vi "Sample Data Demo v1.vi"() -> ()   [LabVIEW 2020]
doc: "Sample data demonstration, also allows to test saving functinoality without having to be conected to the machine."
panel:
  out "output cluster 3":cluster{dbl[], dbl[]}
  out "output cluster":cluster{dbl[], dbl[]}
  in  "Tab Control":enum32{"A-Scan", "B-Scan", "C-Scan"}(tab)
  out "A-Scan":cluster{dbl[], dbl[]}(graph)
  in  "Folder to Save Data":path
  in  "File Name":string
  in  "Confirm Saving Options":bool
  in  "A Scan Scan":bool
  in  "Desired 'Y' Position":dbl
  in  "Desired 'X' Position":dbl
  in  "File Format":T1(radio)
  in  "B-Scan File Name":string
  in  "Folder to Save B-Scan Data":path
  out "B-Scan":dbl[][](graph)
  in  "Depth Along Axis":dbl
  in  "Position of Selected Axis":dbl
  in  "B Scan Scan":bool
  in  "Confirm Saving Options 2":bool
  in  "File Format":T1(radio)
  in  "Folder To Save A-Scan Data":path
  in  "A-Scan File Name":string
  in  "B-Scan Build Up Quality":T2(radio)
  in  "C-Scan Build Up Quantity":T2(radio)
  in  "Total 'Y' Distance to Cover":dbl
  in  "Total 'X' Distance to Cover":dbl
  in  "C Scan Scan":bool
  out "C-Scan":dbl[][](graph)
  in  "File Format":T1(radio)=enum."Do Not Save"
  in  "Confirm Saving Options":bool
  in  "A-Scan File Name":string
  in  "Folder to Save A-Scan Data":path
  in  "Folder to Save C-Scan Data":path
  in  "C-Scan File Name":string
  # "Scan Parameters"
  # "Saving Options"
  # "Scan Parameters"
  # "Saving Options"
  # "Scan Parameters"
  # "Saving Options"
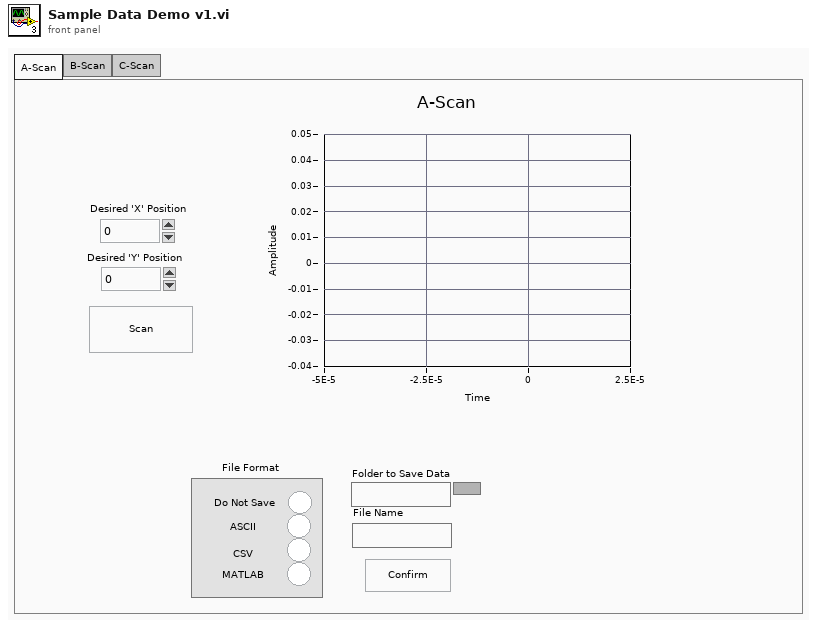
[diagram p1: front panel]
types:
  T1 = enum32{"No Selection", "Do Not Save", "ASCII", "CSV", "MATLAB"}
  T2 = enum32{"No Selection", "Peak Positive", "Peak Negative", "Peak Magnitude", "Energy"}
  T3 = enum16{"open", "replace", "create", "open or create", "replace or create", "replace or create with confirmation"}
  T4 = enum8{"Enabled", "Disabled", "Disabled and Grayed Out"}
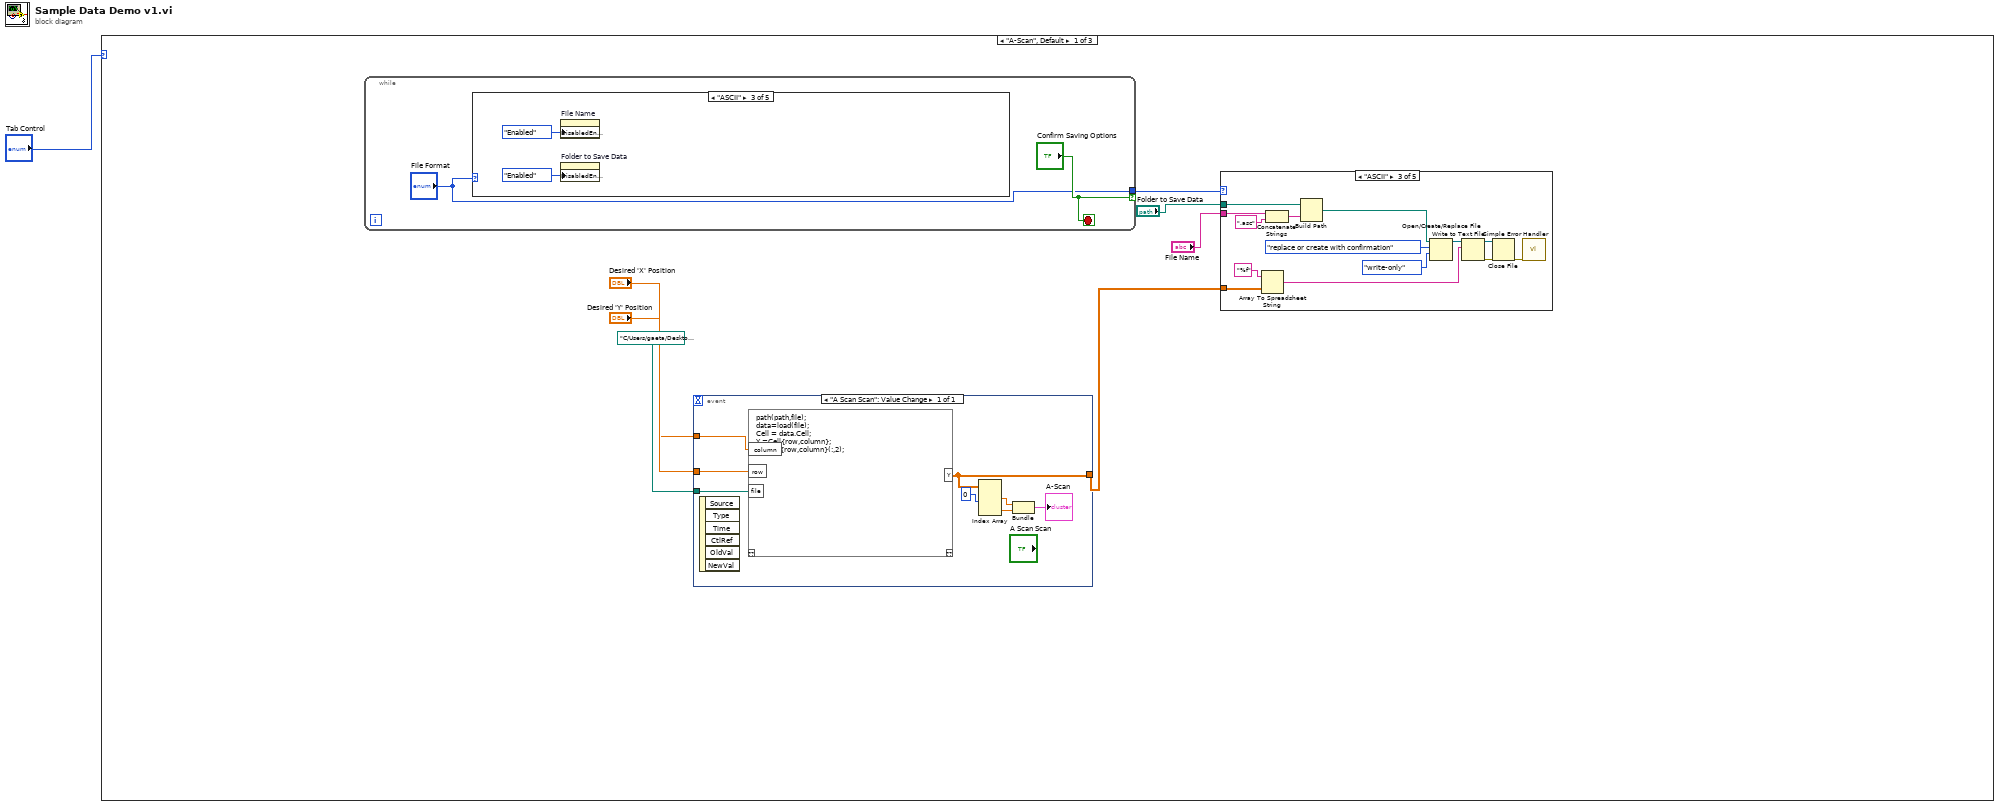
[diagram p0: block diagram]
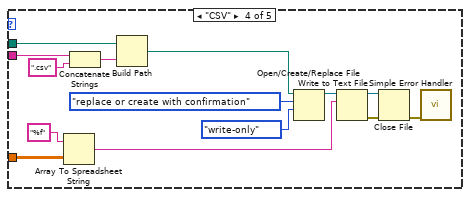
[diagram p4: hidden frame]
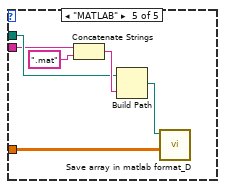
[diagram p5: hidden frame]
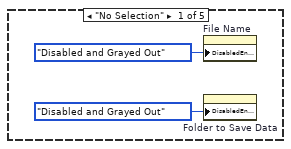
[diagram p6: hidden frame]
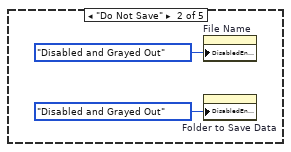
[diagram p7: hidden frame]
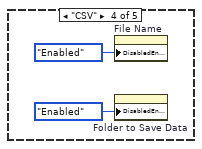
[diagram p8: hidden frame]
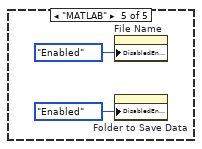
[diagram p9: hidden frame]
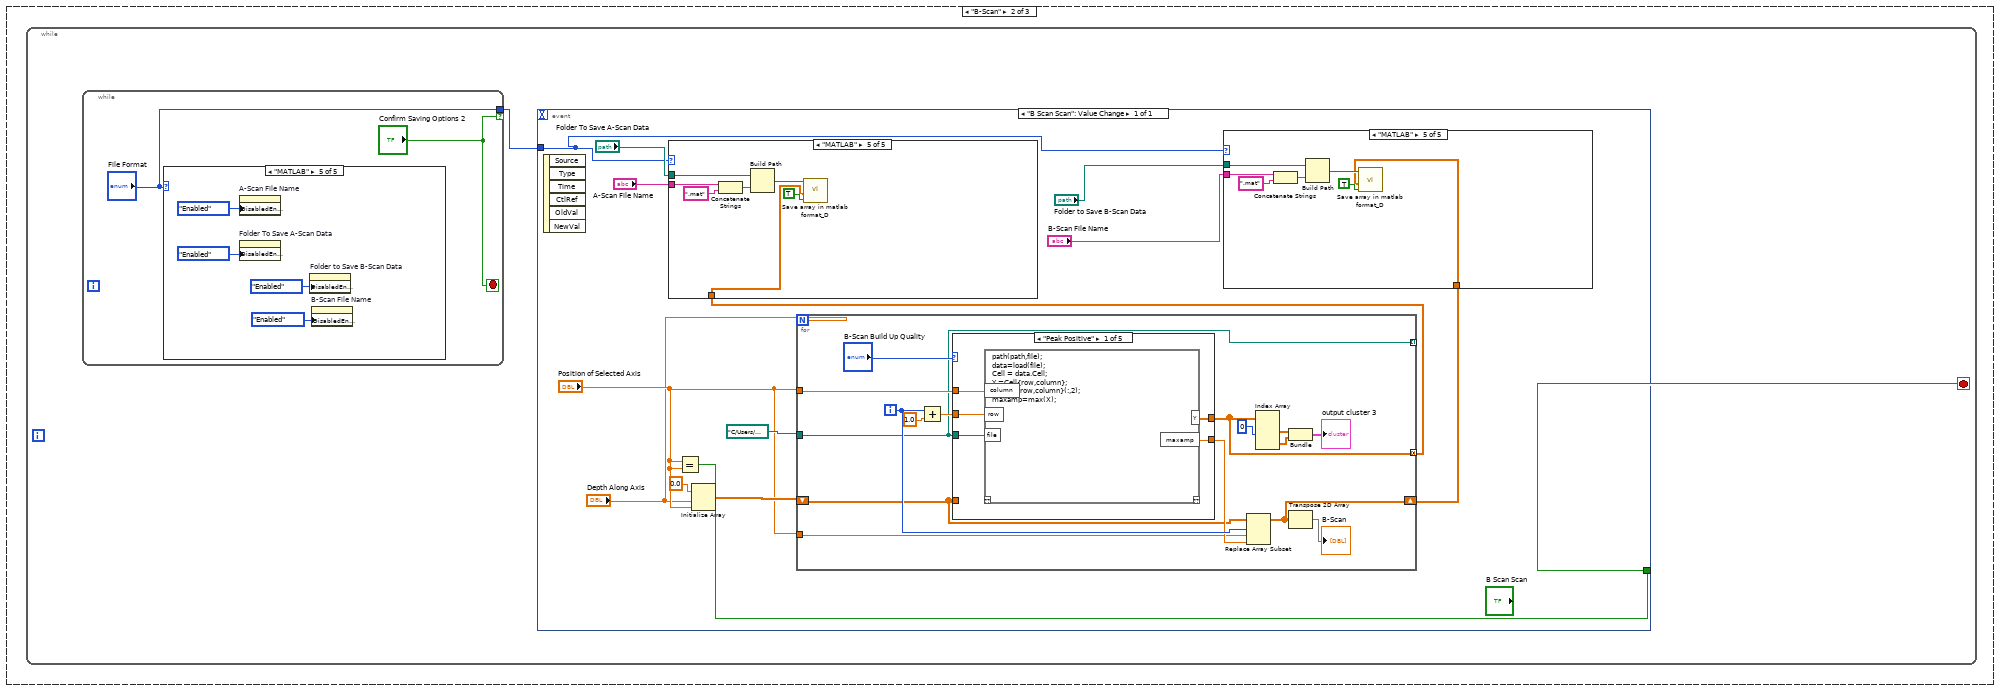
[diagram p10: hidden frame]
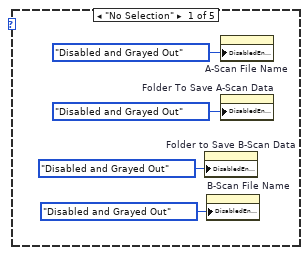
[diagram p11: hidden frame]
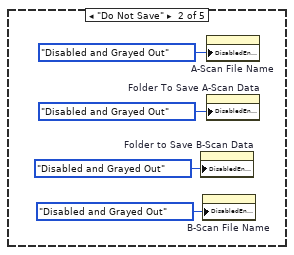
[diagram p12: hidden frame]
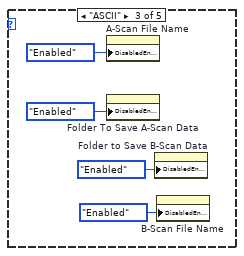
[diagram p13: hidden frame]
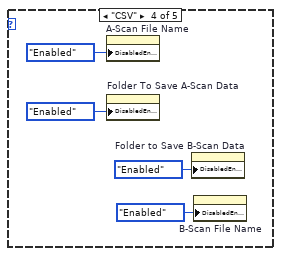
[diagram p14: hidden frame]
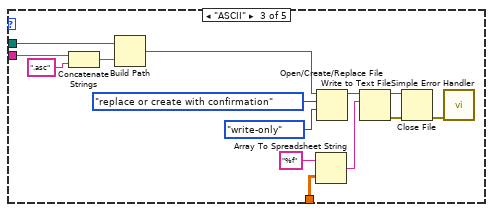
[diagram p17: hidden frame]
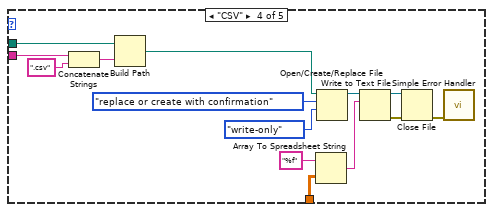
[diagram p18: hidden frame]
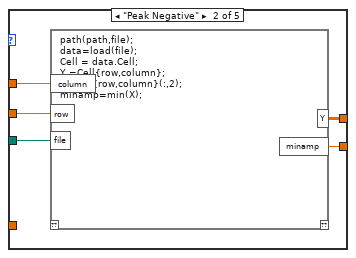
[diagram p19: hidden frame]
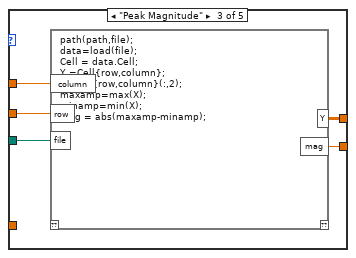
[diagram p20: hidden frame]
diagram:
  n1 = case shown="\"A-Scan\", Default" "Tab Control" {
    frame "A-Scan", Default {
      n2 = while {
        tunnel: ["File Format"] -> w2 if="Confirm Saving Options"
        stop <- "Confirm Saving Options" stop-if-true
        n3 = case shown="\"ASCII\"" "File Format" {
          frame "No Selection" {
            n4 = property on="File Name" class="Str"("DisabledEnum"=T4."Disabled and Grayed Out" ("Disabled")) -> ()  [unwired: 2 in, 2 out]
            n5 = property on="Folder to Save Data" class="Path"("DisabledEnum"=T4."Disabled and Grayed Out" ("Disabled")) -> ()  [unwired: 2 in, 2 out]
          }
          frame "Do Not Save" {
            n6 = property on="File Name" class="Str"("DisabledEnum"=T4."Disabled and Grayed Out" ("Disabled")) -> ()  [unwired: 2 in, 2 out]
            n7 = property on="Folder to Save Data" class="Path"("DisabledEnum"=T4."Disabled and Grayed Out" ("Disabled")) -> ()  [unwired: 2 in, 2 out]
          }
          frame "ASCII" {
            n8 = property on="File Name" class="Str"("DisabledEnum"=T4."Enabled" ("Disabled")) -> ()  [unwired: 2 in, 2 out]
            n9 = property on="Folder to Save Data" class="Path"("DisabledEnum"=T4."Enabled" ("Disabled")) -> ()  [unwired: 2 in, 2 out]
          }
          frame "CSV" {
            n10 = property on="File Name" class="Str"("DisabledEnum"=T4."Enabled" ("Disabled")) -> ()  [unwired: 2 in, 2 out]
            n11 = property on="Folder to Save Data" class="Path"("DisabledEnum"=T4."Enabled" ("Disabled")) -> ()  [unwired: 2 in, 2 out]
          }
          frame "MATLAB" {
            n12 = property on="File Name" class="Str"("DisabledEnum"=T4."Enabled" ("Disabled")) -> ()  [unwired: 2 in, 2 out]
            n13 = property on="Folder to Save Data" class="Path"("DisabledEnum"=T4."Enabled" ("Disabled")) -> ()  [unwired: 2 in, 2 out]
          }
        }
      }
      n14 = event shown="[0] \"A Scan Scan\": Value Change" {
        selector: _ -> [_]
        dyn-events: _ -> [_]
        timeout: _ -> [_]
        tunnel: "Desired 'X' Position" -> [w56]
        tunnel: "Desired 'Y' Position" -> [w58]
        tunnel: path "C:/Users/gaeta/Desktop/Unif Leerstof/Individual Project/Osc. Data/wetransfer-86c2d3/2DZXaxisscan 0.28MHz 30x30mm 20mvpp 1020L centre 390mm from td plane.mat" ("Input Data Path") -> [w57]
        tunnel: [w55] -> w5
        event "A Scan Scan": Value Change {
          n15 = event-data() -> ()  [unwired: 1 in, 6 out]
          n16 = script code="path(path,file);\ndata=load(file);\nCell = data.Cell;\nY =Cell{row,column};\nX=Cell{row,column}(:,2);"("row"=w58, "file"=w57, "column"=w56) -> ("Y"=w55:dbl[][])  [unwired: 1 in, 1 out]
          n17 = Index Array(array=w55, index (col) #1=0 ("disabled index (col)")) -> (element #1=w61:dbl[], element #2=w60:dbl[])  [unwired: 3 in]
          n18 = Bundle(w61, w60) -> (→"A-Scan":cluster{dbl[], dbl[]})  [unwired: 1 in]
        }
      }
      n19 = case shown="\"ASCII\"" w2 {
        tunnel: w5 -> [_ _ w9 w25 w37]
        tunnel: "Folder to Save Data" -> [_ _ w11 w24 w39]
        tunnel: "File Name" -> [_ _ w10 w23 w38]
        frame "No Selection" {
        }
        frame "Do Not Save" {
        }
        frame "ASCII" {
          n20 = Array To Spreadsheet String(array=w9, 3:"%f" ("format string")) -> (spreadsheet string=w21:string)  [unwired: 1 in]
          n21 = Concatenate Strings(w10, ".asc" ("string")) -> (w16:string)
          n22 = Build Path(base path=w11, name or relative path=w16) -> (appended path=w17:path)
          n23 = Open/Create/Replace File(file path (use dialog)=w17, operation (0:open)=T3."replace or create with confirmation", access (0:read/write)=enum16{"read/write", "read-only", "write-only"}."write-only") -> (refnum out=w22:refnum<file>)  [unwired: 1 in, 4 out]
          n24 = Write to Text File(file (use dialog)=w22, text=w21) -> (refnum out=w20:refnum<file>, error out=w19:errorcluster)  [unwired: 2 in, 1 out]
          n25 = Close File(refnum=w20, error in=w19) -> (error out=w18:errorcluster)  [unwired: 1 out]
          n26 = call <vilib>:"Simple Error Handler.vi"("error in (no error)"=w18) -> ()  [unwired: 1 in, 8 out]
        }
        frame "CSV" {
          n27 = Array To Spreadsheet String(array=w25, 3:"%f" ("format string")) -> (spreadsheet string=w32:string)  [unwired: 1 in]
          n28 = Concatenate Strings(w23, ".csv" ("string")) -> (w31:string)
          n29 = Build Path(base path=w24, name or relative path=w31) -> (appended path=w30:path)
          n30 = Open/Create/Replace File(file path (use dialog)=w30, operation (0:open)=T3."replace or create with confirmation", access (0:read/write)=enum16{"read/write", "read-only", "write-only"}."write-only") -> (refnum out=w36:refnum<file>)  [unwired: 1 in, 4 out]
          n31 = Write to Text File(file (use dialog)=w36, text=w32) -> (refnum out=w33:refnum<file>, error out=w34:errorcluster)  [unwired: 2 in, 1 out]
          n32 = Close File(refnum=w33, error in=w34) -> (error out=w35:errorcluster)  [unwired: 1 out]
          n33 = call <vilib>:"Simple Error Handler.vi"("error in (no error)"=w35) -> ()  [unwired: 1 in, 8 out]
        }
        frame "MATLAB" {
          n34 = Concatenate Strings(w38, ".mat" ("string")) -> (w41:string)
          n35 = Build Path(base path=w39, name or relative path=w41) -> (appended path=w42:path)
          n36 = call "Save array in matlab format_D"("2D array"=w37, "file path (dialog if empty)"=w42) -> ()  [unwired: 5 in, 1 out]
        }
      }
    }
    frame "B-Scan" {
      n37 = while {
        stop <- w64 stop-if-true
        n38 = while {
          tunnel: ["File Format"] -> w63 if="Confirm Saving Options 2"
          stop <- "Confirm Saving Options 2" stop-if-true
          n39 = case shown="\"MATLAB\"" "File Format" {
            frame "No Selection" {
              n40 = property on="Folder to Save B-Scan Data" class="Path"("DisabledEnum"=T4."Disabled and Grayed Out" ("Disabled")) -> ()  [unwired: 2 in, 2 out]
              n41 = property on="B-Scan File Name" class="Str"("DisabledEnum"=T4."Disabled and Grayed Out" ("Disabled")) -> ()  [unwired: 2 in, 2 out]
              n42 = property on="A-Scan File Name" class="Str"("DisabledEnum"=T4."Disabled and Grayed Out" ("Disabled")) -> ()  [unwired: 2 in, 2 out]
              n43 = property on="Folder To Save A-Scan Data" class="Path"("DisabledEnum"=T4."Disabled and Grayed Out" ("Disabled")) -> ()  [unwired: 2 in, 2 out]
            }
            frame "Do Not Save" {
              n44 = property on="Folder to Save B-Scan Data" class="Path"("DisabledEnum"=T4."Disabled and Grayed Out" ("Disabled")) -> ()  [unwired: 2 in, 2 out]
              n45 = property on="B-Scan File Name" class="Str"("DisabledEnum"=T4."Disabled and Grayed Out" ("Disabled")) -> ()  [unwired: 2 in, 2 out]
              n46 = property on="A-Scan File Name" class="Str"("DisabledEnum"=T4."Disabled and Grayed Out" ("Disabled")) -> ()  [unwired: 2 in, 2 out]
              n47 = property on="Folder To Save A-Scan Data" class="Path"("DisabledEnum"=T4."Disabled and Grayed Out" ("Disabled")) -> ()  [unwired: 2 in, 2 out]
            }
            frame "ASCII" {
              n48 = property on="A-Scan File Name" class="Str"("DisabledEnum"=T4."Enabled" ("Disabled")) -> ()  [unwired: 2 in, 2 out]
              n49 = property on="Folder To Save A-Scan Data" class="Path"("DisabledEnum"=T4."Enabled" ("Disabled")) -> ()  [unwired: 2 in, 2 out]
              n50 = property on="Folder to Save B-Scan Data" class="Path"("DisabledEnum"=T4."Enabled" ("Disabled")) -> ()  [unwired: 2 in, 2 out]
              n51 = property on="B-Scan File Name" class="Str"("DisabledEnum"=T4."Enabled" ("Disabled")) -> ()  [unwired: 2 in, 2 out]
            }
            frame "CSV" {
              n52 = property on="A-Scan File Name" class="Str"("DisabledEnum"=T4."Enabled" ("Disabled")) -> ()  [unwired: 2 in, 2 out]
              n53 = property on="Folder To Save A-Scan Data" class="Path"("DisabledEnum"=T4."Enabled" ("Disabled")) -> ()  [unwired: 2 in, 2 out]
              n54 = property on="Folder to Save B-Scan Data" class="Path"("DisabledEnum"=T4."Enabled" ("Disabled")) -> ()  [unwired: 2 in, 2 out]
              n55 = property on="B-Scan File Name" class="Str"("DisabledEnum"=T4."Enabled" ("Disabled")) -> ()  [unwired: 2 in, 2 out]
            }
            frame "MATLAB" {
              n56 = property on="A-Scan File Name" class="Str"("DisabledEnum"=T4."Enabled" ("Disabled")) -> ()  [unwired: 2 in, 2 out]
              n57 = property on="Folder To Save A-Scan Data" class="Path"("DisabledEnum"=T4."Enabled" ("Disabled")) -> ()  [unwired: 2 in, 2 out]
              n58 = property on="Folder to Save B-Scan Data" class="Path"("DisabledEnum"=T4."Enabled" ("Disabled")) -> ()  [unwired: 2 in, 2 out]
              n59 = property on="B-Scan File Name" class="Str"("DisabledEnum"=T4."Enabled" ("Disabled")) -> ()  [unwired: 2 in, 2 out]
            }
          }
        }
        n60 = event shown="[0] \"B Scan Scan\": Value Change" {
          selector: _ -> [_]
          dyn-events: _ -> [_]
          timeout: _ -> [_]
          tunnel: [w92] -> w64
          tunnel: w63 -> [w87]
          event "B Scan Scan": Value Change {
            n61 = event-data() -> ()  [unwired: 1 in, 6 out]
            n62 = Equal?(x="Position of Selected Axis", y="Position of Selected Axis") -> (x = y?=w92:bool)
            n63 = Initialize Array(0.0 ("element"), "Depth Along Axis", "Position of Selected Axis") -> (w95:dbl[][])
            n64 = for {
              N: "Depth Along Axis" -> [_]
              tunnel: [w136] -> _ mode=indexing
              tunnel: "Position of Selected Axis" -> [w144]
              shift-right: [w145] -> w88
              shift-left: w95 -> [w141]
              tunnel: [w137] -> w93 mode=concatenating
              tunnel: path "C:/Users/gaeta/Desktop/Unif Leerstof/Individual Project/Osc. Data/wetransfer-86c2d3/2DZXaxisscan 0.28MHz 30x30mm 20mvpp 1020L centre 390mm from td plane.mat" ("Input Data Path") -> [w136]
              tunnel: "Position of Selected Axis" -> [w135]
              i -> [w146]
              n65 = Add(x=w146, y=1.0) -> (x+y=w143:dbl)
              n66 = case shown="\"Peak Positive\"" "B-Scan Build Up Quality" {
                tunnel: w144 -> [w151 w156 w161 w166 _]
                tunnel: w143 -> [w155 w160 w163 w168 _]
                tunnel: w136 -> [w154 w159 w162 w167 _]
                tunnel: [w152 w158 w164 w169 _] -> w142
                tunnel: [w153 w157 w165 w170 _] -> w137
                tunnel: w141 -> [_ _ _ _ _]
                frame "Peak Positive" {
                  n67 = script code="path(path,file);\ndata=load(file);\nCell = data.Cell;\nY =Cell{row,column};\nX=Cell{row,column}(:,2);\nmaxamp=max(X);"("row"=w155, "file"=w154, "column"=w151) -> ("Y"=w153:dbl[][], "maxamp"=w152:dbl)  [unwired: 1 in, 1 out]
                }
                frame "Peak Negative" {
                  n68 = script code="path(path,file);\ndata=load(file);\nCell = data.Cell;\nY =Cell{row,column};\nX=Cell{row,column}(:,2);\nminamp=min(X);"("row"=w160, "file"=w159, "column"=w156) -> ("Y"=w157:dbl[][], "minamp"=w158:dbl)  [unwired: 1 in, 1 out]
                }
                frame "Peak Magnitude" {
                  n69 = script code="path(path,file);\ndata=load(file);\nCell = data.Cell;\nY =Cell{row,column};\nX=Cell{row,column}(:,2);\nmaxamp=max(X);\nminamp=min(X);\nmag = abs(maxamp-minamp);"("row"=w163, "file"=w162, "column"=w161) -> ("Y"=w165:dbl[][], "mag"=w164:dbl)  [unwired: 1 in, 1 out]
                }
                frame "Energy" {
                  n70 = script code="path(path,file);\ndata=load(file);\nCell = data.Cell;\nY =Cell{row,column};\nX=Cell{row,column}(:,2);\narea=trapz(X);"("row"=w168, "file"=w167, "column"=w166) -> ("Y"=w170:dbl[][], "area"=w169:dbl)  [unwired: 1 in, 1 out]
                }
                frame "No Selection" {
                }
              }
              n71 = Replace Array Subset(array=w141, new element=w142, index (row)=w146, index (col)=w135) -> (w145:dbl[][])
              n72 = Index Array(array=w137, index (col) #1=0 ("disabled index (col)")) -> (element #1=w148:dbl[], element #2=w149:dbl[])  [unwired: 3 in]
              n73 = Bundle(w148, w149) -> (→"output cluster 3":cluster{dbl[], dbl[]})  [unwired: 1 in]
              n74 = Transpose 2D Array(2D array=w145) -> (transposed array=→"B-Scan":dbl[][])
            }
            n75 = case shown="\"MATLAB\"" w87 {
              tunnel: "Folder To Save A-Scan Data" -> [_ _ w173 w187 w202]
              tunnel: "A-Scan File Name" -> [_ _ w172 w186 w201]
              tunnel: w93 -> [_ _ w171 w185 w199]
              frame "No Selection" {
              }
              frame "Do Not Save" {
              }
              frame "ASCII" {
                n76 = Concatenate Strings(w172, ".asc" ("string")) -> (w178:string)
                n77 = Build Path(base path=w173, name or relative path=w178) -> (appended path=w179:path)
                n78 = Array To Spreadsheet String(array=w171, 3:"%f" ("format string")) -> (spreadsheet string=w183:string)  [unwired: 1 in]
                n79 = Open/Create/Replace File(file path (use dialog)=w179, operation (0:open)=T3."replace or create with confirmation", access (0:read/write)=enum16{"read/write", "read-only", "write-only"}."write-only") -> (refnum out=w184:refnum<file>)  [unwired: 1 in, 4 out]
                n80 = Write to Text File(file (use dialog)=w184, text=w183) -> (refnum out=w182:refnum<file>, error out=w181:errorcluster)  [unwired: 2 in, 1 out]
                n81 = Close File(refnum=w182, error in=w181) -> (error out=w180:errorcluster)  [unwired: 1 out]
                n82 = call <vilib>:"Simple Error Handler.vi"("error in (no error)"=w180) -> ()  [unwired: 1 in, 8 out]
              }
              frame "CSV" {
                n83 = Concatenate Strings(w186, ".csv" ("string")) -> (w193:string)
                n84 = Build Path(base path=w187, name or relative path=w193) -> (appended path=w192:path)
                n85 = Array To Spreadsheet String(array=w185, 3:"%f" ("format string")) -> (spreadsheet string=w194:string)  [unwired: 1 in]
                n86 = Open/Create/Replace File(file path (use dialog)=w192, operation (0:open)=T3."replace or create with confirmation", access (0:read/write)=enum16{"read/write", "read-only", "write-only"}."write-only") -> (refnum out=w198:refnum<file>)  [unwired: 1 in, 4 out]
                n87 = Write to Text File(file (use dialog)=w198, text=w194) -> (refnum out=w195:refnum<file>, error out=w196:errorcluster)  [unwired: 2 in, 1 out]
                n88 = Close File(refnum=w195, error in=w196) -> (error out=w197:errorcluster)  [unwired: 1 out]
                n89 = call <vilib>:"Simple Error Handler.vi"("error in (no error)"=w197) -> ()  [unwired: 1 in, 8 out]
              }
              frame "MATLAB" {
                n90 = Concatenate Strings(w201, ".mat" ("string")) -> (w204:string)
                n91 = Build Path(base path=w202, name or relative path=w204) -> (appended path=w205:path)
                n92 = call "Save array in matlab format_D"("append to file? (new file:F)"=TRUE, "2D array"=w199, "file path (dialog if empty)"=w205) -> ()  [unwired: 4 in, 1 out]
              }
            }
            n93 = case shown="\"MATLAB\"" w87 {
              tunnel: "Folder to Save B-Scan Data" -> [_ _ w102 w116 w131]
              tunnel: "B-Scan File Name" -> [_ _ w101 w115 w130]
              tunnel: w88 -> [_ _ w100 w114 w128]
              frame "No Selection" {
              }
              frame "Do Not Save" {
              }
              frame "ASCII" {
                n94 = Concatenate Strings(w101, ".asc" ("string")) -> (w107:string)
                n95 = Build Path(base path=w102, name or relative path=w107) -> (appended path=w108:path)
                n96 = Array To Spreadsheet String(array=w100, 3:"%f" ("format string")) -> (spreadsheet string=w112:string)  [unwired: 1 in]
                n97 = Open/Create/Replace File(file path (use dialog)=w108, operation (0:open)=T3."replace or create with confirmation", access (0:read/write)=enum16{"read/write", "read-only", "write-only"}."write-only") -> (refnum out=w113:refnum<file>)  [unwired: 1 in, 4 out]
                n98 = Write to Text File(file (use dialog)=w113, text=w112) -> (refnum out=w111:refnum<file>, error out=w110:errorcluster)  [unwired: 2 in, 1 out]
                n99 = Close File(refnum=w111, error in=w110) -> (error out=w109:errorcluster)  [unwired: 1 out]
                n100 = call <vilib>:"Simple Error Handler.vi"("error in (no error)"=w109) -> ()  [unwired: 1 in, 8 out]
              }
              frame "CSV" {
                n101 = Concatenate Strings(w115, ".csv" ("string")) -> (w122:string)
                n102 = Build Path(base path=w116, name or relative path=w122) -> (appended path=w121:path)
                n103 = Array To Spreadsheet String(array=w114, 3:"%f" ("format string")) -> (spreadsheet string=w123:string)  [unwired: 1 in]
                n104 = Open/Create/Replace File(file path (use dialog)=w121, operation (0:open)=T3."replace or create with confirmation", access (0:read/write)=enum16{"read/write", "read-only", "write-only"}."write-only") -> (refnum out=w127:refnum<file>)  [unwired: 1 in, 4 out]
                n105 = Write to Text File(file (use dialog)=w127, text=w123) -> (refnum out=w124:refnum<file>, error out=w125:errorcluster)  [unwired: 2 in, 1 out]
                n106 = Close File(refnum=w124, error in=w125) -> (error out=w126:errorcluster)  [unwired: 1 out]
                n107 = call <vilib>:"Simple Error Handler.vi"("error in (no error)"=w126) -> ()  [unwired: 1 in, 8 out]
              }
              frame "MATLAB" {
                n108 = Concatenate Strings(w130, ".mat" ("string")) -> (w133:string)
                n109 = Build Path(base path=w131, name or relative path=w133) -> (appended path=w134:path)
                n110 = call "Save array in matlab format_D"("append to file? (new file:F)"=TRUE, "2D array"=w128, "file path (dialog if empty)"=w134) -> ()  [unwired: 4 in, 1 out]
              }
            }
          }
        }
      }
    }
    frame "C-Scan" {
      n111 = while {
        stop <- w207 stop-if-true
        n112 = while {
          tunnel: ["File Format"] -> w206 if="Confirm Saving Options"
          stop <- "Confirm Saving Options" stop-if-true
          n113 = case shown="\"ASCII\"" "File Format" {
            frame "No Selection" {
              n114 = property on="Folder to Save C-Scan Data" class="Path"("DisabledEnum"=T4."Disabled and Grayed Out" ("Disabled")) -> ()  [unwired: 2 in, 2 out]
              n115 = property on="A-Scan File Name" class="Str"("DisabledEnum"=T4."Disabled and Grayed Out" ("Disabled")) -> ()  [unwired: 2 in, 2 out]
              n116 = property on="Folder to Save A-Scan Data" class="Path"("DisabledEnum"=T4."Disabled and Grayed Out" ("Disabled")) -> ()  [unwired: 2 in, 2 out]
              n117 = property on="C-Scan File Name" class="Str"("DisabledEnum"=T4."Disabled and Grayed Out" ("Disabled")) -> ()  [unwired: 2 in, 2 out]
            }
            frame "Do Not Save" {
              n118 = property on="A-Scan File Name" class="Str"("DisabledEnum"=T4."Disabled and Grayed Out" ("Disabled")) -> ()  [unwired: 2 in, 2 out]
              n119 = property on="Folder to Save A-Scan Data" class="Path"("DisabledEnum"=T4."Disabled and Grayed Out" ("Disabled")) -> ()  [unwired: 2 in, 2 out]
              n120 = property on="Folder to Save C-Scan Data" class="Path"("DisabledEnum"=T4."Disabled and Grayed Out" ("Disabled")) -> ()  [unwired: 2 in, 2 out]
              n121 = property on="C-Scan File Name" class="Str"("DisabledEnum"=T4."Disabled and Grayed Out" ("Disabled")) -> ()  [unwired: 2 in, 2 out]
            }
            frame "ASCII" {
              n122 = property on="A-Scan File Name" class="Str"("DisabledEnum"=T4."Enabled" ("Disabled")) -> ()  [unwired: 2 in, 2 out]
              n123 = property on="Folder to Save A-Scan Data" class="Path"("DisabledEnum"=T4."Enabled" ("Disabled")) -> ()  [unwired: 2 in, 2 out]
              n124 = property on="Folder to Save C-Scan Data" class="Path"("DisabledEnum"=T4."Enabled" ("Disabled")) -> ()  [unwired: 2 in, 2 out]
              n125 = property on="C-Scan File Name" class="Str"("DisabledEnum"=T4."Enabled" ("Disabled")) -> ()  [unwired: 2 in, 2 out]
            }
            frame "CSV" {
              n126 = property on="A-Scan File Name" class="Str"("DisabledEnum"=T4."Enabled" ("Disabled")) -> ()  [unwired: 2 in, 2 out]
              n127 = property on="Folder to Save A-Scan Data" class="Path"("DisabledEnum"=T4."Enabled" ("Disabled")) -> ()  [unwired: 2 in, 2 out]
              n128 = property on="Folder to Save C-Scan Data" class="Path"("DisabledEnum"=T4."Enabled" ("Disabled")) -> ()  [unwired: 2 in, 2 out]
              n129 = property on="C-Scan File Name" class="Str"("DisabledEnum"=T4."Enabled" ("Disabled")) -> ()  [unwired: 2 in, 2 out]
            }
            frame "MATLAB" {
              n130 = property on="A-Scan File Name" class="Str"("DisabledEnum"=T4."Enabled" ("Disabled")) -> ()  [unwired: 2 in, 2 out]
              n131 = property on="Folder to Save A-Scan Data" class="Path"("DisabledEnum"=T4."Enabled" ("Disabled")) -> ()  [unwired: 2 in, 2 out]
              n132 = property on="Folder to Save C-Scan Data" class="Path"("DisabledEnum"=T4."Enabled" ("Disabled")) -> ()  [unwired: 2 in, 2 out]
              n133 = property on="C-Scan File Name" class="Str"("DisabledEnum"=T4."Enabled" ("Disabled")) -> ()  [unwired: 2 in, 2 out]
            }
          }
        }
        n134 = event shown="[0] \"C Scan Scan\": Value Change" {
          selector: _ -> [_]
          dyn-events: _ -> [_]
          timeout: _ -> [_]
          tunnel: [w239] -> w207
          tunnel: [w231] -> _
          tunnel: [w238] -> _
          tunnel: w206 -> [w230]
          event "C Scan Scan": Value Change {
            n135 = event-data() -> ()  [unwired: 1 in, 6 out]
            n136 = Initialize Array(0.0 ("element"), "Total 'Y' Distance to Cover", "Total 'X' Distance to Cover") -> (w242:dbl[][])
            n137 = for {
              N: "Total 'X' Distance to Cover" -> [_]
              tunnel: path "C:/Users/gaeta/Desktop/Unif Leerstof/Individual Project/Osc. Data/wetransfer-86c2d3/2DZXaxisscan 0.28MHz 30x30mm 20mvpp 1020L centre 390mm from td plane.mat" ("Input Data Path") -> [w323]
              tunnel: "Total 'Y' Distance to Cover" -> [w321]
              shift-right: [w319] -> w231
              shift-left: w242 -> [w320]
              tunnel: [w317] -> w240
              tunnel: [w316] -> w238 mode=indexing
              tunnel: [w315] -> w234 mode=concatenating
              i -> [w318]
              n138 = Add(x=w318, y=1.0) -> (x+y=w317:dbl)
              n139 = for {
                N: w321 -> [_]
                tunnel: w323 -> [w330]
                tunnel: w317 -> [w332]
                shift-right: [w334] -> w319
                shift-left: w320 -> [w328]
                tunnel: w318 -> [w333]
                tunnel: [w325] -> w316 mode=indexing
                tunnel: [w325] -> w315 mode=concatenating
                i -> [w335]
                n140 = Add(x=w335, y=1.0) -> (x+y=w331:dbl)
                n141 = case shown="\"Energy\"" "C-Scan Build Up Quantity" {
                  tunnel: w332 -> [w340 w345 w350 w355 _]
                  tunnel: w331 -> [w344 w349 w352 w357 _]
                  tunnel: w330 -> [w343 w348 w351 w356 _]
                  tunnel: [w341 w347 w353 w358 _] -> w329
                  tunnel: [w342 w346 w354 w359 _] -> w325
                  tunnel: w328 -> [_ _ _ _ _]
                  frame "Peak Positive" {
                    n142 = script code="path(path,file);\ndata=load(file);\nCell = data.Cell;\nY =Cell{row,column};\nX=Cell{row,column}(:,2);\nmaxamp=max(X);"("row"=w344, "file"=w343, "column"=w340) -> ("Y"=w342:dbl[][], "maxamp"=w341:dbl)  [unwired: 1 in, 1 out]
                  }
                  frame "Peak Negative" {
                    n143 = script code="path(path,file);\ndata=load(file);\nCell = data.Cell;\nY =Cell{row,column};\nX=Cell{row,column}(:,2);\nminamp=min(X);"("row"=w349, "file"=w348, "column"=w345) -> ("Y"=w346:dbl[][], "minamp"=w347:dbl)  [unwired: 1 in, 1 out]
                  }
                  frame "Peak Magnitude" {
                    n144 = script code="path(path,file);\ndata=load(file);\nCell = data.Cell;\nY =Cell{row,column};\nX=Cell{row,column}(:,2);\nmaxamp=max(X);\nminamp=min(X);\nmag = abs(maxamp-minamp);"("row"=w352, "file"=w351, "column"=w350) -> ("Y"=w354:dbl[][], "mag"=w353:dbl)  [unwired: 1 in, 1 out]
                  }
                  frame "Energy" {
                    n145 = script code="path(path,file);\ndata=load(file);\nCell = data.Cell;\nY =Cell{row,column};\nX=Cell{row,column}(:,2);\narea=trapz(X);"("row"=w357, "file"=w356, "column"=w355) -> ("Y"=w359:dbl[][], "area"=w358:dbl)  [unwired: 1 in, 1 out]
                  }
                  frame "No Selection" {
                  }
                }
                n146 = Replace Array Subset(array=w328, new element=w329, index (row)=w335, index (col)=w333) -> (w334:dbl[][])
                n147 = Index Array(array=w325, index (col) #1=0 ("disabled index (col)")) -> (element #1=w337:dbl[], element #2=w338:dbl[])  [unwired: 3 in]
                n148 = Bundle(w337, w338) -> (→"output cluster":cluster{dbl[], dbl[]})  [unwired: 1 in]
                n149 = Transpose 2D Array(2D array=w334) -> (transposed array=→"C-Scan":dbl[][])
              }
            }
            n150 = Equal?(x=w240, y="Total 'X' Distance to Cover") -> (x = y?=w239:bool)
            n151 = case shown="\"MATLAB\"" w230 {
              tunnel: "Folder to Save C-Scan Data" -> [_ _ w247 w261 w276]
              tunnel: "C-Scan File Name" -> [_ _ w246 w260 w275]
              tunnel: w231 -> [_ _ w245 w259 w273]
              frame "No Selection" {
              }
              frame "Do Not Save" {
              }
              frame "ASCII" {
                n152 = Array To Spreadsheet String(array=w245, 3:"%f" ("format string")) -> (spreadsheet string=w257:string)  [unwired: 1 in]
                n153 = Concatenate Strings(w246, ".asc" ("string")) -> (w252:string)
                n154 = Build Path(base path=w247, name or relative path=w252) -> (appended path=w253:path)
                n155 = Open/Create/Replace File(file path (use dialog)=w253, operation (0:open)=T3."replace or create with confirmation", access (0:read/write)=enum16{"read/write", "read-only", "write-only"}."write-only") -> (refnum out=w258:refnum<file>)  [unwired: 1 in, 4 out]
                n156 = Write to Text File(file (use dialog)=w258, text=w257) -> (refnum out=w256:refnum<file>, error out=w255:errorcluster)  [unwired: 2 in, 1 out]
                n157 = Close File(refnum=w256, error in=w255) -> (error out=w254:errorcluster)  [unwired: 1 out]
                n158 = call <vilib>:"Simple Error Handler.vi"("error in (no error)"=w254) -> ()  [unwired: 1 in, 8 out]
              }
              frame "CSV" {
                n159 = Array To Spreadsheet String(array=w259, 3:"%f" ("format string")) -> (spreadsheet string=w268:string)  [unwired: 1 in]
                n160 = Concatenate Strings(w260, ".csv" ("string")) -> (w267:string)
                n161 = Build Path(base path=w261, name or relative path=w267) -> (appended path=w266:path)
                n162 = Open/Create/Replace File(file path (use dialog)=w266, operation (0:open)=T3."replace or create with confirmation", access (0:read/write)=enum16{"read/write", "read-only", "write-only"}."write-only") -> (refnum out=w272:refnum<file>)  [unwired: 1 in, 4 out]
                n163 = Write to Text File(file (use dialog)=w272, text=w268) -> (refnum out=w269:refnum<file>, error out=w270:errorcluster)  [unwired: 2 in, 1 out]
                n164 = Close File(refnum=w269, error in=w270) -> (error out=w271:errorcluster)  [unwired: 1 out]
                n165 = call <vilib>:"Simple Error Handler.vi"("error in (no error)"=w271) -> ()  [unwired: 1 in, 8 out]
              }
              frame "MATLAB" {
                n166 = Concatenate Strings(w275, ".mat" ("string")) -> (w278:string)
                n167 = Build Path(base path=w276, name or relative path=w278) -> (appended path=w279:path)
                n168 = call "Save array in matlab format_D"("append to file? (new file:F)"=TRUE, "2D array"=w273, "file path (dialog if empty)"=w279) -> ()  [unwired: 4 in, 1 out]
              }
            }
            n169 = case shown="\"ASCII\"" w230 {
              tunnel: "Folder to Save A-Scan Data" -> [_ _ w282 w296 w311]
              tunnel: "A-Scan File Name" -> [_ _ w281 w295 w310]
              tunnel: w234 -> [_ _ w280 w294 w308]
              frame "No Selection" {
              }
              frame "Do Not Save" {
              }
              frame "ASCII" {
                n170 = Array To Spreadsheet String(array=w280, 3:"%f" ("format string")) -> (spreadsheet string=w292:string)  [unwired: 1 in]
                n171 = Concatenate Strings(w281, ".asc" ("string")) -> (w287:string)
                n172 = Build Path(base path=w282, name or relative path=w287) -> (appended path=w288:path)
                n173 = Open/Create/Replace File(file path (use dialog)=w288, operation (0:open)=T3."replace or create with confirmation", access (0:read/write)=enum16{"read/write", "read-only", "write-only"}."write-only") -> (refnum out=w293:refnum<file>)  [unwired: 1 in, 4 out]
                n174 = Write to Text File(file (use dialog)=w293, text=w292) -> (refnum out=w291:refnum<file>, error out=w290:errorcluster)  [unwired: 2 in, 1 out]
                n175 = Close File(refnum=w291, error in=w290) -> (error out=w289:errorcluster)  [unwired: 1 out]
                n176 = call <vilib>:"Simple Error Handler.vi"("error in (no error)"=w289) -> ()  [unwired: 1 in, 8 out]
              }
              frame "CSV" {
                n177 = Array To Spreadsheet String(array=w294, 3:"%f" ("format string")) -> (spreadsheet string=w303:string)  [unwired: 1 in]
                n178 = Concatenate Strings(w295, ".csv" ("string")) -> (w302:string)
                n179 = Build Path(base path=w296, name or relative path=w302) -> (appended path=w301:path)
                n180 = Open/Create/Replace File(file path (use dialog)=w301, operation (0:open)=T3."replace or create with confirmation", access (0:read/write)=enum16{"read/write", "read-only", "write-only"}."write-only") -> (refnum out=w307:refnum<file>)  [unwired: 1 in, 4 out]
                n181 = Write to Text File(file (use dialog)=w307, text=w303) -> (refnum out=w304:refnum<file>, error out=w305:errorcluster)  [unwired: 2 in, 1 out]
                n182 = Close File(refnum=w304, error in=w305) -> (error out=w306:errorcluster)  [unwired: 1 out]
                n183 = call <vilib>:"Simple Error Handler.vi"("error in (no error)"=w306) -> ()  [unwired: 1 in, 8 out]
              }
              frame "MATLAB" {
                n184 = Concatenate Strings(w310, ".mat" ("string")) -> (w313:string)
                n185 = Build Path(base path=w311, name or relative path=w313) -> (appended path=w314:path)
                n186 = call "Save array in matlab format_D"("append to file? (new file:F)"=TRUE, "2D array"=w308, "file path (dialog if empty)"=w314) -> ()  [unwired: 4 in, 1 out]
              }
            }
          }
        }
      }
    }
  }
